vi "welcome.vi"(8 "error in (no error)":errorcluster, 11 "simonMessages in":refnum<class "simonMessages.lvclass">) -> (0 "error out":errorcluster, 3 "simonMessages out":refnum<class "simonMessages.lvclass">)   [LabVIEW 2019, in "simonMessages.lvclass"]
uses:
  simonMessages.lvclass
  simonMessages.lvclass/simonMessages.ctl
  TextDisplay/TextDisplay Class.lvclass
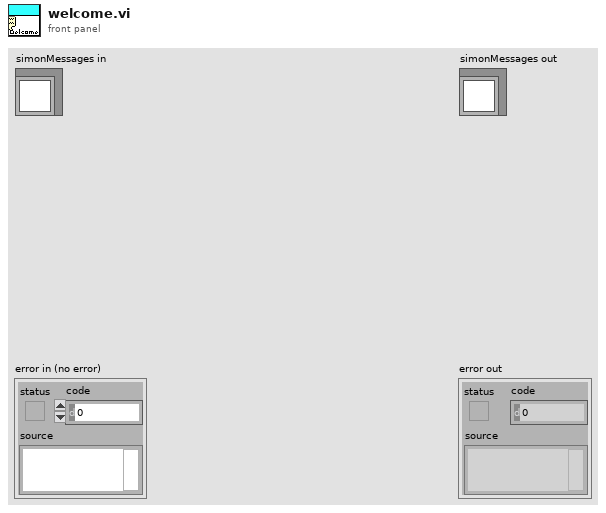
[diagram p1: front panel]
types:
  T1 = cluster{"Text":string, "Size":u8, "Justification":enum16{"Left", "Center", "Right"}, "Display Type":string}
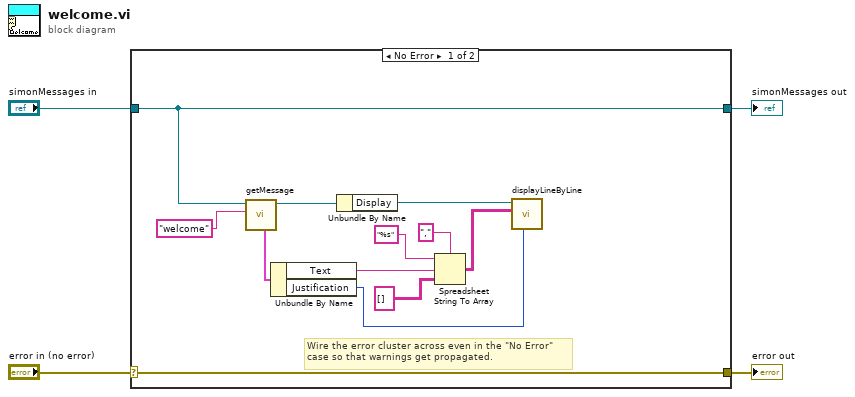
[diagram p0: block diagram]
diagram:
  n1 = case shown="No Error" "error in (no error)" {
    selector: "error in (no error)" -> [w16 w18]
    tunnel: [w16 w18] -> w3
    tunnel: [w14 w17] -> w1
    tunnel: "simonMessages in" -> [w14 w17]
    frame No Error {
      # "Wire the error cluster across even in the \"No Error\"\ncase so that warnings get propagated."
      n2 = call "getMessage.vi"("key"="welcome", "simonMessages in"=w14) -> ("Message Cluster"=w10:T1, "simonMessages out"=w13:refnum<class "simonMessages.lvclass">)  [unwired: 7 in, 1 out]
      n3 = Unbundle By Name(w10) -> ("Text"=w6:string, "Justification"=w5:enum16{"Left", "Center", "Right"})
      n4 = Unbundle By Name(w13) -> ("Display"=w15:refnum<class "TextDisplay Class.lvclass">)
      n5 = Spreadsheet String To Array(delimiter (Tab)=",", format string="%s", spreadsheet string=w6, array type (2D Dbl)=string[][] []) -> (array=w8:string[][])
      n6 = call "displayLineByLine.vi"("Justification"=w5, "scoreLog"=w8, "TextDisplay Class in"=w15) -> ()  [unwired: 7 in, 2 out]
    }
    frame Error {
    }
  }
  "error out" <- w3
  "simonMessages out" <- w1
